vi "HV507 Set All Low.vi"(8 "Error In":errorcluster, 11 "LINX Resource In":T1) -> (0 "Error Out":errorcluster, 3 "LINX Resource Out":T1)   [LabVIEW 2017]
doc: "Pulls all HV outputs from HV507 low by writing 0 to the ~BL (blanking) pin number 29.\n\nThis VI requires that the Arduino DIO pin 7 is tied to ~BL on HV507."
uses:
  <vilib>/MakerHub/LINX/Private/Type Defs/LINX Ref.ctl
  <vilib>/MakerHub/LINX/Private/Type Defs/Platform.ctl
  <vilib>/MakerHub/LINX/Private/Type Defs/Interface.ctl
  <vilib>/MakerHub/LINX/Private/Device/Type Defs/LINX Device Config.ctl
  <vilib>/MakerHub/LINX/Private/Device/Type Defs/TCP Config.ctl
  <vilib>/MakerHub/LINX/Private/Device/Type Defs/Channels.ctl
  <vilib>/MakerHub/LINX/Public/Peripherals/Digital/Digital Write 1 Chan.vi
  <vilib>/MakerHub/LINX/Public/Peripherals/Digital/Digital Write N Chans.vi
  <vilib>/MakerHub/LINX/Private/Local IO/LinxDigitalWrite.vi
  <vilib>/MakerHub/LINX/Public/Utilities/Check Channel.vi
  <vilib>/MakerHub/LINX/Private/Utilties/Generate Error.vi
  <vilib>/MakerHub/LINX/LMH-LINX.lvlib
  <vilib>/MakerHub/LINX/Private/Device/Device.lvlib
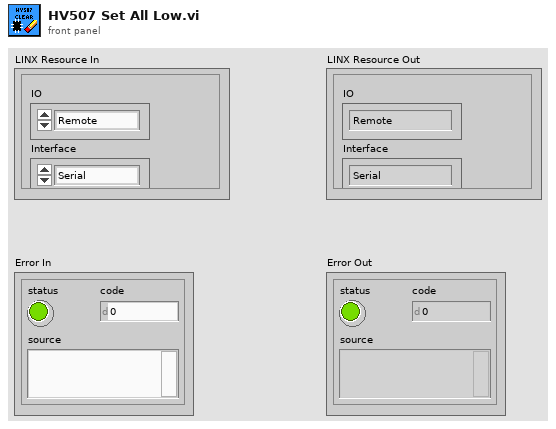
[diagram p1: front panel]
types:
  T1 = typedef "LMH-LINX.lvlib/LINX Ref.ctl" = cluster{"IO":T2, "Interface":T3, "LINX Device Config":T4}
  T2 = typedef "LMH-LINX.lvlib/Platform.ctl" = enum16{"Remote", "Local"}
  T3 = typedef "LMH-LINX.lvlib/Interface.ctl" = enum16{"Serial", "TCP"}
  T4 = typedef "LMH-LINX.lvlib/Device.lvlib/LINX Device Config.ctl" = cluster{"Interface":T3, "COM Port":refnum<visa-resource-name>, "TCP Configuration":T5, "Device Family":u8, "Device ID":u8, "Device Name":string, "TCP Ref":refnum<k5>, "Channels":T6}
  T5 = typedef "LMH-LINX.lvlib/Device.lvlib/TCP Config.ctl" = cluster{"IP Address":string, "Port":u16}
  T6 = typedef "LMH-LINX.lvlib/Channels.ctl" = cluster{"DI":u8[], "DO":u8[], "AI":u8[], "AO":u8[], "PWM":u8[], "QE":u8[], "UART":u8[], "I2C 2":u8[], "SPI":u8[], "CAN":u8[], "Servo":u8[], "AI Ref (V)":dbl, "AI Resolution (Bits)":u8, "AO Ref (V)":dbl, "AO Resolution (Bits)":u8}
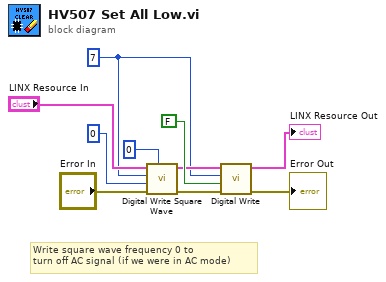
[diagram p0: block diagram]
diagram:
  w4 = u8 7 ("DO Channel")
  # "Write square wave frequency 0 to\nturn off AC signal (if we were in AC mode)"
  n1 = call <vilib>:"Digital Write Square Wave.vi"("Duration (ms)"=u32 0, "Error In"="Error In", "Frequency (Hz)"=u32 0, "Channel"=w4, "LINX Resource"="LINX Resource In") -> ("Error Out"=w5:errorcluster, "LINX Resource"=w6:T1)  [unwired: 5 in]
  n2 = call-poly <vilib>:"Digital Write.vi"("Error In"=w5, "Output Value"=FALSE, "DO Channel"=w4, "LINX Resource"=w6) -> ("Error Out"=→"Error Out":errorcluster, "LINX Resource"=→"LINX Resource Out":T1)  [unwired: 6 in]
